vi "Get Key Value (Double Array).vi"(5 "Key name":string, 6 "Default value":dbl[](array[numeric]), 7 "Section name":string, 8 "error in (no error)":errorcluster, 9 "Use LV Default? [F]":bool, 11 "Carya Config in":refnum<class "Carya Config.lvclass">) -> (0 "error out":errorcluster, 1 "Found?":bool, 2 "value":dbl[](array[numeric]), 3 "Carya Config out":refnum<class "Carya Config.lvclass">)   [LabVIEW 2013, in "Carya Config.lvclass"]
doc: "Copyright 2018, Carya Automatisering, Wiebe Walstra."
uses:
  Carya Config.lvclass
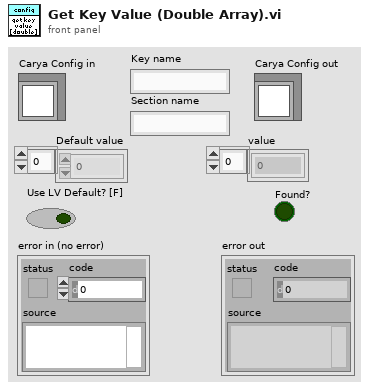
[diagram p1: front panel]
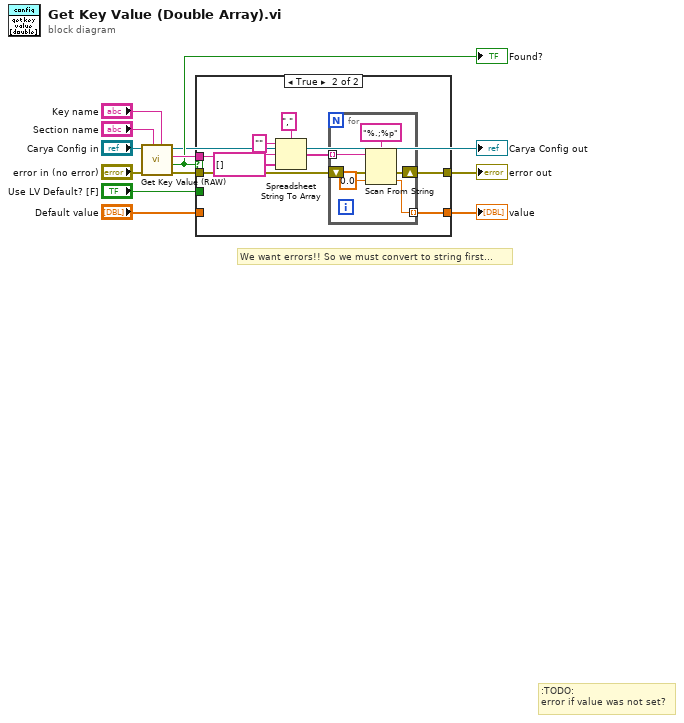
[diagram p0: block diagram]
diagram:
  # "We want errors!! So we must convert to string first..."
  # ":TODO:\nerror if value was not set?"
  n1 = call-dynamic "Get Key Value (RAW).vi"("Key name"="Key name", "Section name"="Section name", "error in (no error)"="error in (no error)", "Carya Config in"="Carya Config in") -> ("error out"=w11:errorcluster, "Found?"=w4:bool, "Value"=w6:string, "Carya Config out"=→"Carya Config out":refnum<class "Carya Config.lvclass">)  [unwired: 4 in]
  "Found?" <- w4
  n2 = case shown="True" w4 {
    tunnel: w11 -> [w13 w18]
    tunnel: [w13 w15] -> w7
    tunnel: w6 -> [_ w17]
    tunnel: "Default value" -> [w14 _]
    tunnel: [w14 w16] -> w3
    tunnel: "Use LV Default? [F]" -> [_ _]
    frame False {
    }
    frame True {
      n3 = Spreadsheet String To Array(delimiter (Tab)=",", format string="", spreadsheet string=w17, array type (2D Dbl)=string[] []) -> (array=w19:string[])
      n4 = for {
        tunnel: w19 -> [w28] mode=indexing
        tunnel: [w25] -> w16 mode=indexing
        shift-right: [w23] -> w15
        shift-left: w18 -> [w24]
        n5 = Scan From String(format string="%.;%p", input string=w28, error in=w24, default 1=0.0 ("default value 1")) -> (error out=w23:errorcluster, output 1=w25:dbl)  [unwired: 1 in, 2 out]
      }
    }
  }
  "error out" <- w7
  "value" <- w3
